vi "Set Resource.vi"(8 "error in (no error)":errorcluster, 10 "Resource":refnum<class "Resource.lvclass">, 11 "Device in":refnum<class "Device.lvclass">) -> (0 "error out":errorcluster, 3 "Device out":refnum<class "Device.lvclass">)   [LabVIEW 2020, in "PicoG-App.lvlib" / "Device.lvclass"]
uses:
  Device.lvclass
  Builds/picoG/ppl/PicoG-Core.lvlibp/PicoG-Processor/PicoG-Core/DeployResource/Resource.lvclass
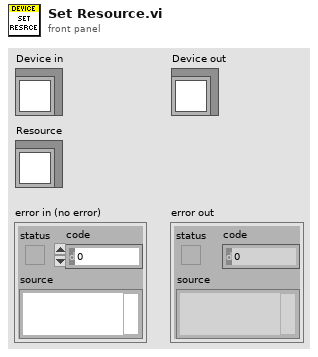
[diagram p1: front panel]
types:
  T1 = typedef "PicoG-App.lvlib/Device.lvclass/Resource Ref.ctl" = cluster{"Resource":refnum<class "Resource.lvclass">, "Open":bool, "At Prompt":bool, "Running":bool}
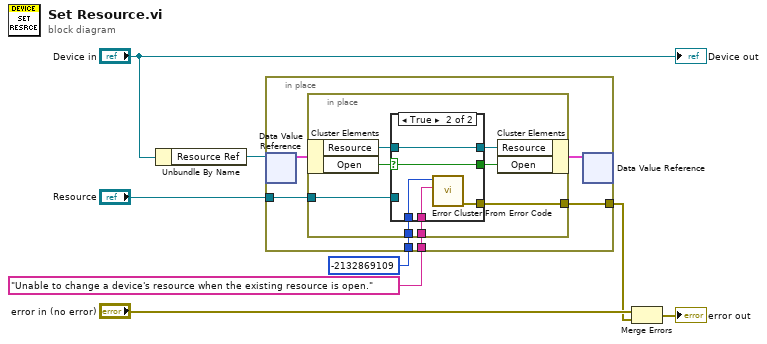
[diagram p0: block diagram]
diagram:
  n1 = Unbundle By Name("Device in") -> ("Resource Ref"=w7:refnum<data-value>)
  n2 = in-place {
    in-place-border: "Resource" -> [w12]
    in-place-border: [w11] -> w3
    in-place-border: -2132869109 -> [w10]
    in-place-border: "Unable to change a device's resource when the existing resource is open." -> [w9]
    n3 = in-place-dvr #1(w7) -> (w14:T1)  [unwired: 1 out]
    n4 = in-place {
      in-place-border: w12 -> [w18]
      in-place-border: [w17] -> w11
      in-place-border: w10 -> [w16]
      in-place-border: w9 -> [w15]
      n5 = in-place-cluster #2(w14) -> ("Resource"=w21:refnum<class "Resource.lvclass">, "Open"=w22:bool)
      n6 = case shown="True" w22 {
        selector: w22 -> [_ w25]
        tunnel: w21 -> [_ w24]
        tunnel: [w23 w24] -> w20
        tunnel: [_ w25] -> w19
        tunnel: w18 -> [w23 _]
        tunnel: [_ w27] -> w17
        tunnel: w16 -> [_ w28]
        tunnel: w15 -> [_ w26]
        frame False {
        }
        frame True {
          n7 = call <vilib>:"Error Cluster From Error Code.vi"("error message (\"\")"=w26, "error code (0)"=w28) -> ("error out"=w27:errorcluster)  [unwired: 7 in]
        }
      }
      n8 = in-place-cluster #2("Resource"=w20, "Open"=w19) -> (w13:T1)
    }
    n9 = in-place-dvr #1(w13) -> ()  [unwired: 2 out]
  }
  n10 = Merge Errors("error in (no error)", w3) -> (→"error out":errorcluster)
  "Device out" <- "Device in"
